vi "Array 1.vi"() -> ()   [LabVIEW 2011]
panel:
  out "Subset":dbl[](array[numeric])
  in  "Length":dbl
  in  "Index":dbl
  in  "Input Array":dbl[](array[numeric])
  out "Array 3":dbl[](array[numeric])
  in  "Numeric":dbl
  in  "Array 2":dbl[](array[numeric])
  out "Sorted Array":dbl[](array[numeric])
  in  "Array":dbl[](array[numeric])
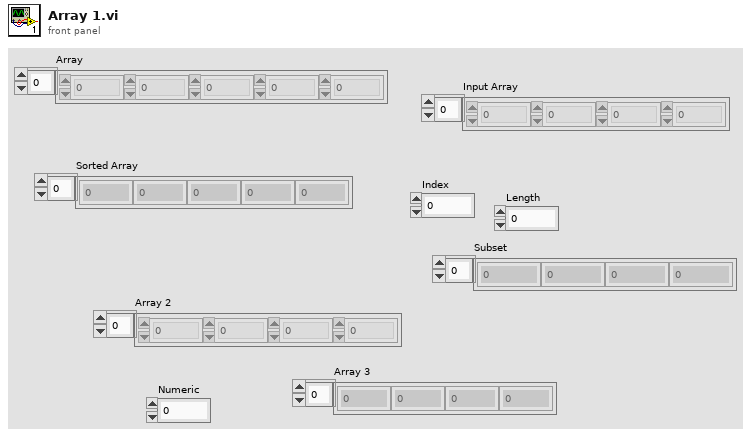
[diagram p1: front panel]
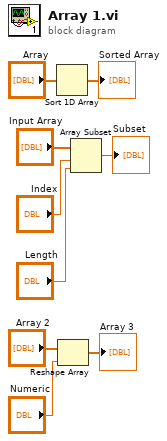
[diagram p0: block diagram]
diagram:
  n1 = Sort 1D Array(array="Array") -> (sorted array=→"Sorted Array":dbl[])
  n2 = Reshape Array("Array 2", "Numeric") -> (→"Array 3":dbl[])
  n3 = Array Subset(array="Input Array", index="Index", length="Length") -> (→"Subset":dbl[])
